vi "set_context.vi"(7 "context":string, 8 "error in (no error)":errorcluster, 11 "File Log Provider in":refnum<class "File Log Provider.lvclass">) -> (0 "error out":errorcluster, 3 "File Log Provider out":refnum<class "File Log Provider.lvclass">)   [LabVIEW 2019, in "File Log Provider.lvclass"]
uses:
  File Log Provider.lvclass
  Queue Log Provider/Queue Log Provider.lvclass
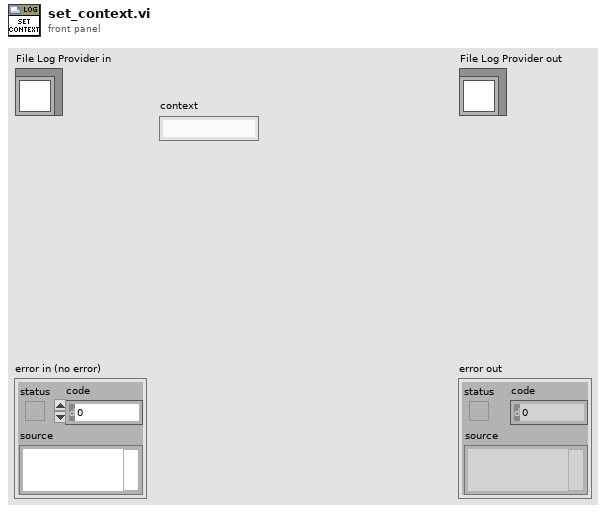
[diagram p1: front panel]
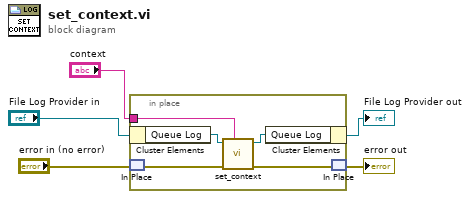
[diagram p0: block diagram]
diagram:
  n1 = in-place {
    in-place-border: "context" -> [w8]
    n2 = in-place-cluster #1("File Log Provider in") -> ("Queue Log"=w10:refnum<class "Queue Log Provider.lvclass">)
    n3 = in-place-match #2("error in (no error)") -> (w7:errorcluster)
    n4 = call-dynamic "set_context.vi"("context"=w8, "error in (no error)"=w7, "Queue Log Provider in"=w10) -> ("error out"=w6:errorcluster, "Queue Log Provider out"=w9:refnum<class "Queue Log Provider.lvclass">)  [unwired: 7 in]
    n5 = in-place-cluster #1("Queue Log"=w9) -> (→"File Log Provider out":refnum<class "File Log Provider.lvclass">)
    n6 = in-place-match #2(w6) -> (→"error out":errorcluster)
  }
